vi "Sync Move Arm to.vi"(9 "Speed":dbl=2.0, 11 "Target Position":dbl) -> ()   [LabVIEW 2012]
uses:
  Robot Global Data.vi
  Arm Globals.vi
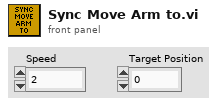
[diagram p1: front panel]
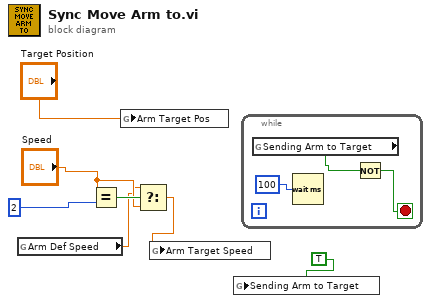
[diagram p0: block diagram]
diagram:
  n1 = global read "Arm Globals.vi" "Arm Def Speed"() -> (w2:dbl)
  n2 = Equal?(x="Speed", y=2) -> (x = y?=w4:bool)
  n3 = global write "Robot Global Data.vi" "Arm Target Pos"("Target Position") -> ()
  n4 = Select(t=w2, s=w4, f="Speed") -> (s? t:f=w1:dbl)
  n5 = global write "Robot Global Data.vi" "Arm Target Speed"(w1) -> ()
  n6 = global write "Robot Global Data.vi" "Sending Arm to Target"(TRUE) -> ()
  n7 = while {
    stop <- w8 stop-if-true
    n8 = global read "Robot Global Data.vi" "Sending Arm to Target"() -> (w9:bool)
    n9 = Wait (ms)(milliseconds to wait=100) -> ()  [unwired: 1 out]
    n10 = Not(x=w9) -> (.not. x?=w8:bool)
  }
